vi "tm_setparameter_a.vi"(6 "Index":i32, 8 "error in (no error)":errorcluster, 9 "Value in":dbl, 10 "Parameter":u32(ring)=4212128 items=["SENSOR MODE"=4212128, "CCD MODE"=4212384, "READOUT MODE"=4211872, "ACTIVE VIEW INDEX"=4343136, "BITS PER CHANNEL"=4342976, "IMAGE PIXEL TYPE"=4343296, "BINNING"=4215968, "EXPOSURE TIME"=2049184, "CONTRAST GAIN"=3163312, "CONTRAST OFFSET"=3163328, "LIGHT MODE"=2114720, "SENSITIVITY"=2114992, "PHOTON IMAGING MODE"=2115200, "HIGH DYNAMIC RANGE MODE"=3163360, "WHITE BALANCE"=3163568, "TEMPERATURE"=2115232, "TEMPERATURE TARGET"=2115264, "SENSOR COOLER FAN"=2115296, "LINEBUNDLE HEIGHT"=4212192, "MECHANICAL SHUTTER"=2115488, "BACK FOCUS POSITION"=8422304, "TRIGGER CONNECTOR"=1066432, "TRIGGER SOURCE"=1066144, "OUTPUT TRIGGER SOURCE"=1852576, "TRIGGER GLOBAL EXPOSURE"=2049680, "FIRST TRIGGER BEHAVIOR"=2049696, "CHANNEL SYNC"=1852352, "READOUT DIRECTION"=4211904, "PRE HSYNC COUNT"=1852704, "INTERNAL LINE SPEED"=4226000, "INTERNAL LINE INTERVAL"=4226016], 11 "Handle in":u32) -> (0 "error out":errorcluster, 3 "Handle out":u32)   [LabVIEW 2012]
uses:
  tmcamcon.dll
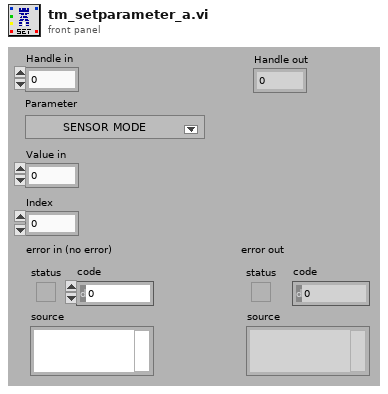
[diagram p1: front panel]
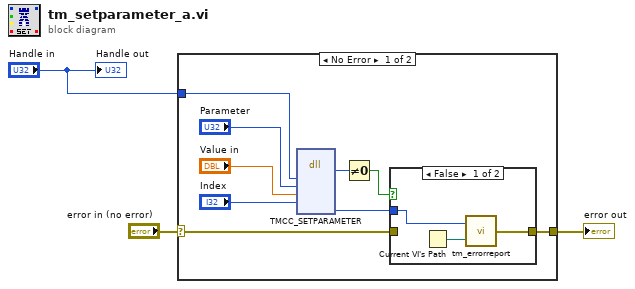
[diagram p0: block diagram]
diagram:
  n1 = case shown="No Error" "error in (no error)" {
    selector: "error in (no error)" -> [w7 w17]
    tunnel: [w4 w17] -> w2
    tunnel: "Handle in" -> [w8 _]
    frame No Error {
      n2 = dll-call lib="tmcamcon.dll" fn="TMCC_SETPARAMETER"("HDCAM"=w8, "parameter"="Parameter", "value"="Value in", "view"="Index") -> ("return type"=w12:u32, "Erval"=w6:i32)  [unwired: 8 in, 2 out]
      n3 = Not Equal To 0?(x=w12) -> (x != 0?=w5:bool)
      n4 = case shown="False" w5 {
        tunnel: w7 -> [_ w16]
        tunnel: [w14 w16] -> w4
        tunnel: w6 -> [w13 _]
        frame False {
          n5 = Current VI's Path() -> (path=w15:path)
          n6 = call "tm_errorreport.vi"("Source"=w15, "Error"=w13) -> ("error out"=w14:errorcluster)
        }
        frame True {
        }
      }
    }
    frame Error {
    }
  }
  "error out" <- w2
  "Handle out" <- "Handle in"
